vi "Version_4.9_8_on-chip_valves_for25ulSyringe_withModfied_Plunging.vi"() -> ()   [LabVIEW 2020] (continued)
                                n7542 = call "HardStopCurrentProcess (SubVI).vi"("VISA Refnum in"=w7985) -> ()  [unwired: 11 in]
                                }
                              }
                              n7543 = call "ProcessCompletionWaiter (SubVI).vi"("VISA Refnum in"=w7984) -> ()  [unwired: 11 in]
                            }
                            frame #4 {
                              # "Switch to Port-1"
                              # "Port-1 of the pump is conncted to Waste"
                              n7544 = local read "VISA Refnum in\nfor Pump"() -> (w7987:refnum<visa-resource-name>)
                              n7545 = call "PortChanger (SubVI).vi"("Port Number"="1", "VISA Refnum in"=w7987) -> ()  [unwired: 10 in]
                            }
                            frame #5 {
                              n7546 = local read "Stopper that ends \nthe main loops"() -> (w7988:bool)
                              n7547 = local read "VISA Refnum in\nfor Pump"() -> (w7989:refnum<visa-resource-name>)
                              n7548 = case shown="True" w7988 {
                                frame False {
                                }
                                frame True {
                                n7549 = local read "VISA Refnum in\nfor Pump"() -> (w7990:refnum<visa-resource-name>)
                                n7550 = call "HardStopCurrentProcess (SubVI).vi"("VISA Refnum in"=w7990) -> ()  [unwired: 11 in]
                                }
                              }
                              n7551 = call "ProcessCompletionWaiter (SubVI).vi"("VISA Refnum in"=w7989) -> ()  [unwired: 11 in]
                            }
                            frame #6 {
                              n7552 = local read "VISA Refnum in\nfor Pump"() -> (w7995:refnum<visa-resource-name>)
                              n7553 = local read "Volume of Syringe"() -> (w7994:dbl)
                              n7554 = call "GoToAbsolutePosition(SubVI).vi"("Absolute Volume Position in Syringe (in ul)"=0.0 ("Volume to be Dispensed"), "Volume of Syringe"=w7994, "Resolution of Pumping"=T2."Standard Pumping" ("Resolution for Dispensing"), "Flow Rate (ul/min)"=150.0 ("Dispense Flow Rate (ul/min)"), "VISA Refnum in"=w7995) -> ()  [unwired: 6 in, 1 out]
                            }
                            frame #7 {
                              n7555 = local read "Stopper that ends \nthe main loops"() -> (w7997:bool)
                              n7556 = case shown="True" w7997 {
                                frame False {
                                }
                                frame True {
                                n7557 = local read "VISA Refnum in\nfor Pump"() -> (w7998:refnum<visa-resource-name>)
                                n7558 = call "HardStopCurrentProcess (SubVI).vi"("VISA Refnum in"=w7998) -> ()  [unwired: 11 in]
                                }
                              }
                              n7559 = local read "VISA Refnum in\nfor Pump"() -> (w7996:refnum<visa-resource-name>)
                              n7560 = call "ProcessCompletionWaiter (SubVI).vi"("VISA Refnum in"=w7996) -> ()  [unwired: 11 in]
                            }
                          }
                        }
                      }
                      frame #1 {
                        n7561 = local read "No. of \ncleaning cycles"() -> (w7999:i32)
                        n7562 = for {
                          N: w7999 -> [_]
                          n7563 = stacked-sequence {
                            frame #0 {
                              # "Switch to Port-4"
                              # "Port-4 of pump is connected to Buffer-A"
                              n7564 = local read "VISA Refnum in\nfor Pump"() -> (w8002:refnum<visa-resource-name>)
                              n7565 = local write "Pause Data Collection"(TRUE ("Pause Data Collection")) -> ()
                              n7566 = call "PortChanger (SubVI).vi"("Port Number"="4", "VISA Refnum in"=w8002) -> ()  [unwired: 10 in]
                            }
                            frame #1 {
                              n7567 = local read "VISA Refnum in\nfor Pump"() -> (w8003:refnum<visa-resource-name>)
                              n7568 = call "ProcessCompletionWaiter (SubVI).vi"("VISA Refnum in"=w8003) -> ()  [unwired: 11 in]
                            }
                            frame #2 {
                              n7569 = local read "VISA Refnum in\nfor Pump"() -> (w8008:refnum<visa-resource-name>)
                              n7570 = local read "Apparent Volume\nof Syringe"() -> (w8004:dbl)
                              n7571 = local read "Volume of Syringe"() -> (w8007:dbl)
                              n7572 = call "RPickUp(SubVI).vi"("Volume to be picked up"=w8004, "Volume of Syringe"=w8007, "Resolution of PickUP"=T2."Standard Pumping", "PickUp Flow Rate (ul/min)"=150.0, "VISA Refnum in"=w8008) -> ()  [unwired: 6 in, 1 out]
                            }
                            frame #3 {
                              n7573 = local read "Stopper that ends \nthe main loops"() -> (w8009:bool)
                              n7574 = local read "VISA Refnum in\nfor Pump"() -> (w8010:refnum<visa-resource-name>)
                              n7575 = case shown="True" w8009 {
                                frame False {
                                }
                                frame True {
                                n7576 = local read "VISA Refnum in\nfor Pump"() -> (w8011:refnum<visa-resource-name>)
                                n7577 = call "HardStopCurrentProcess (SubVI).vi"("VISA Refnum in"=w8011) -> ()  [unwired: 11 in]
                                }
                              }
                              n7578 = call "ProcessCompletionWaiter (SubVI).vi"("VISA Refnum in"=w8010) -> ()  [unwired: 11 in]
                            }
                            frame #4 {
                              # "Switch to Port-1"
                              # "Port-1 of the pump is conncted to Waste"
                              n7579 = local read "VISA Refnum in\nfor Pump"() -> (w8013:refnum<visa-resource-name>)
                              n7580 = call "PortChanger (SubVI).vi"("Port Number"="1", "VISA Refnum in"=w8013) -> ()  [unwired: 10 in]
                            }
                            frame #5 {
                              n7581 = local read "Stopper that ends \nthe main loops"() -> (w8014:bool)
                              n7582 = local read "VISA Refnum in\nfor Pump"() -> (w8015:refnum<visa-resource-name>)
                              n7583 = case shown="True" w8014 {
                                frame False {
                                }
                                frame True {
                                n7584 = local read "VISA Refnum in\nfor Pump"() -> (w8016:refnum<visa-resource-name>)
                                n7585 = call "HardStopCurrentProcess (SubVI).vi"("VISA Refnum in"=w8016) -> ()  [unwired: 11 in]
                                }
                              }
                              n7586 = call "ProcessCompletionWaiter (SubVI).vi"("VISA Refnum in"=w8015) -> ()  [unwired: 11 in]
                            }
                            frame #6 {
                              n7587 = local read "VISA Refnum in\nfor Pump"() -> (w8021:refnum<visa-resource-name>)
                              n7588 = local read "Volume of Syringe"() -> (w8020:dbl)
                              n7589 = call "GoToAbsolutePosition(SubVI).vi"("Absolute Volume Position in Syringe (in ul)"=0.0 ("Volume to be Dispensed"), "Volume of Syringe"=w8020, "Resolution of Pumping"=T2."Standard Pumping" ("Resolution for Dispensing"), "Flow Rate (ul/min)"=150.0 ("Dispense Flow Rate (ul/min)"), "VISA Refnum in"=w8021) -> ()  [unwired: 6 in, 1 out]
                            }
                            frame #7 {
                              n7590 = local read "Stopper that ends \nthe main loops"() -> (w8023:bool)
                              n7591 = case shown="True" w8023 {
                                frame False {
                                }
                                frame True {
                                n7592 = local read "VISA Refnum in\nfor Pump"() -> (w8024:refnum<visa-resource-name>)
                                n7593 = call "HardStopCurrentProcess (SubVI).vi"("VISA Refnum in"=w8024) -> ()  [unwired: 11 in]
                                }
                              }
                              n7594 = local read "VISA Refnum in\nfor Pump"() -> (w8022:refnum<visa-resource-name>)
                              n7595 = call "ProcessCompletionWaiter (SubVI).vi"("VISA Refnum in"=w8022) -> ()  [unwired: 11 in]
                            }
                          }
                        }
                      }
                      frame #2 {
                        n7596 = local read "No. of \ncleaning cycles"() -> (w8025:i32)
                        n7597 = for {
                          N: w8025 -> [_]
                          n7598 = stacked-sequence {
                            frame #0 {
                              # "Switch to Port-4"
                              # "Port-4 of pump is connected to Buffer-A"
                              n7599 = local read "VISA Refnum in\nfor Pump"() -> (w8028:refnum<visa-resource-name>)
                              n7600 = local write "Pause Data Collection"(TRUE ("Pause Data Collection")) -> ()
                              n7601 = call "PortChanger (SubVI).vi"("Port Number"="5", "VISA Refnum in"=w8028) -> ()  [unwired: 10 in]
                            }
                            frame #1 {
                              n7602 = local read "VISA Refnum in\nfor Pump"() -> (w8029:refnum<visa-resource-name>)
                              n7603 = call "ProcessCompletionWaiter (SubVI).vi"("VISA Refnum in"=w8029) -> ()  [unwired: 11 in]
                            }
                            frame #2 {
                              n7604 = local read "VISA Refnum in\nfor Pump"() -> (w8034:refnum<visa-resource-name>)
                              n7605 = local read "Apparent Volume\nof Syringe"() -> (w8030:dbl)
                              n7606 = local read "Volume of Syringe"() -> (w8033:dbl)
                              n7607 = call "RPickUp(SubVI).vi"("Volume to be picked up"=w8030, "Volume of Syringe"=w8033, "Resolution of PickUP"=T2."Standard Pumping", "PickUp Flow Rate (ul/min)"=150.0, "VISA Refnum in"=w8034) -> ()  [unwired: 6 in, 1 out]
                            }
                            frame #3 {
                              n7608 = local read "Stopper that ends \nthe main loops"() -> (w8035:bool)
                              n7609 = local read "VISA Refnum in\nfor Pump"() -> (w8036:refnum<visa-resource-name>)
                              n7610 = case shown="True" w8035 {
                                frame False {
                                }
                                frame True {
                                n7611 = local read "VISA Refnum in\nfor Pump"() -> (w8037:refnum<visa-resource-name>)
                                n7612 = call "HardStopCurrentProcess (SubVI).vi"("VISA Refnum in"=w8037) -> ()  [unwired: 11 in]
                                }
                              }
                              n7613 = call "ProcessCompletionWaiter (SubVI).vi"("VISA Refnum in"=w8036) -> ()  [unwired: 11 in]
                            }
                            frame #4 {
                              # "Switch to Port-1"
                              # "Port-1 of the pump is conncted to Waste"
                              n7614 = local read "VISA Refnum in\nfor Pump"() -> (w8039:refnum<visa-resource-name>)
                              n7615 = call "PortChanger (SubVI).vi"("Port Number"="1", "VISA Refnum in"=w8039) -> ()  [unwired: 10 in]
                            }
                            frame #5 {
                              n7616 = local read "Stopper that ends \nthe main loops"() -> (w8040:bool)
                              n7617 = local read "VISA Refnum in\nfor Pump"() -> (w8041:refnum<visa-resource-name>)
                              n7618 = case shown="True" w8040 {
                                frame False {
                                }
                                frame True {
                                n7619 = local read "VISA Refnum in\nfor Pump"() -> (w8042:refnum<visa-resource-name>)
                                n7620 = call "HardStopCurrentProcess (SubVI).vi"("VISA Refnum in"=w8042) -> ()  [unwired: 11 in]
                                }
                              }
                              n7621 = call "ProcessCompletionWaiter (SubVI).vi"("VISA Refnum in"=w8041) -> ()  [unwired: 11 in]
                            }
                            frame #6 {
                              n7622 = local read "VISA Refnum in\nfor Pump"() -> (w8047:refnum<visa-resource-name>)
                              n7623 = local read "Volume of Syringe"() -> (w8046:dbl)
                              n7624 = call "GoToAbsolutePosition(SubVI).vi"("Absolute Volume Position in Syringe (in ul)"=0.0 ("Volume to be Dispensed"), "Volume of Syringe"=w8046, "Resolution of Pumping"=T2."Standard Pumping" ("Resolution for Dispensing"), "Flow Rate (ul/min)"=150.0 ("Dispense Flow Rate (ul/min)"), "VISA Refnum in"=w8047) -> ()  [unwired: 6 in, 1 out]
                            }
                            frame #7 {
                              n7625 = local read "Stopper that ends \nthe main loops"() -> (w8049:bool)
                              n7626 = case shown="True" w8049 {
                                frame False {
                                }
                                frame True {
                                n7627 = local read "VISA Refnum in\nfor Pump"() -> (w8050:refnum<visa-resource-name>)
                                n7628 = call "HardStopCurrentProcess (SubVI).vi"("VISA Refnum in"=w8050) -> ()  [unwired: 11 in]
                                }
                              }
                              n7629 = local read "VISA Refnum in\nfor Pump"() -> (w8048:refnum<visa-resource-name>)
                              n7630 = call "ProcessCompletionWaiter (SubVI).vi"("VISA Refnum in"=w8048) -> ()  [unwired: 11 in]
                            }
                          }
                        }
                      }
                      frame #3 {
                        n7631 = local read "No. of \ncleaning cycles"() -> (w8051:i32)
                        n7632 = for {
                          N: w8051 -> [_]
                          n7633 = stacked-sequence {
                            frame #0 {
                              # "Switch to Port-4"
                              # "Port-4 of pump is connected to Buffer-A"
                              n7634 = local read "VISA Refnum in\nfor Pump"() -> (w8054:refnum<visa-resource-name>)
                              n7635 = local write "Pause Data Collection"(TRUE ("Pause Data Collection")) -> ()
                              n7636 = call "PortChanger (SubVI).vi"("Port Number"="7", "VISA Refnum in"=w8054) -> ()  [unwired: 10 in]
                            }
                            frame #1 {
                              n7637 = local read "VISA Refnum in\nfor Pump"() -> (w8055:refnum<visa-resource-name>)
                              n7638 = call "ProcessCompletionWaiter (SubVI).vi"("VISA Refnum in"=w8055) -> ()  [unwired: 11 in]
                            }
                            frame #2 {
                              n7639 = local read "VISA Refnum in\nfor Pump"() -> (w8060:refnum<visa-resource-name>)
                              n7640 = local read "Apparent Volume\nof Syringe"() -> (w8056:dbl)
                              n7641 = local read "Volume of Syringe"() -> (w8059:dbl)
                              n7642 = call "RPickUp(SubVI).vi"("Volume to be picked up"=w8056, "Volume of Syringe"=w8059, "Resolution of PickUP"=T2."Standard Pumping", "PickUp Flow Rate (ul/min)"=150.0, "VISA Refnum in"=w8060) -> ()  [unwired: 6 in, 1 out]
                            }
                            frame #3 {
                              n7643 = local read "Stopper that ends \nthe main loops"() -> (w8061:bool)
                              n7644 = local read "VISA Refnum in\nfor Pump"() -> (w8062:refnum<visa-resource-name>)
                              n7645 = case shown="True" w8061 {
                                frame False {
                                }
                                frame True {
                                n7646 = local read "VISA Refnum in\nfor Pump"() -> (w8063:refnum<visa-resource-name>)
                                n7647 = call "HardStopCurrentProcess (SubVI).vi"("VISA Refnum in"=w8063) -> ()  [unwired: 11 in]
                                }
                              }
                              n7648 = call "ProcessCompletionWaiter (SubVI).vi"("VISA Refnum in"=w8062) -> ()  [unwired: 11 in]
                            }
                            frame #4 {
                              # "Switch to Port-1"
                              # "Port-1 of the pump is conncted to Waste"
                              n7649 = local read "VISA Refnum in\nfor Pump"() -> (w8065:refnum<visa-resource-name>)
                              n7650 = call "PortChanger (SubVI).vi"("Port Number"="1", "VISA Refnum in"=w8065) -> ()  [unwired: 10 in]
                            }
                            frame #5 {
                              n7651 = local read "Stopper that ends \nthe main loops"() -> (w8066:bool)
                              n7652 = local read "VISA Refnum in\nfor Pump"() -> (w8067:refnum<visa-resource-name>)
                              n7653 = case shown="True" w8066 {
                                frame False {
                                }
                                frame True {
                                n7654 = local read "VISA Refnum in\nfor Pump"() -> (w8068:refnum<visa-resource-name>)
                                n7655 = call "HardStopCurrentProcess (SubVI).vi"("VISA Refnum in"=w8068) -> ()  [unwired: 11 in]
                                }
                              }
                              n7656 = call "ProcessCompletionWaiter (SubVI).vi"("VISA Refnum in"=w8067) -> ()  [unwired: 11 in]
                            }
                            frame #6 {
                              n7657 = local read "VISA Refnum in\nfor Pump"() -> (w8073:refnum<visa-resource-name>)
                              n7658 = local read "Volume of Syringe"() -> (w8072:dbl)
                              n7659 = call "GoToAbsolutePosition(SubVI).vi"("Absolute Volume Position in Syringe (in ul)"=0.0 ("Volume to be Dispensed"), "Volume of Syringe"=w8072, "Resolution of Pumping"=T2."Standard Pumping" ("Resolution for Dispensing"), "Flow Rate (ul/min)"=150.0 ("Dispense Flow Rate (ul/min)"), "VISA Refnum in"=w8073) -> ()  [unwired: 6 in, 1 out]
                            }
                            frame #7 {
                              n7660 = local read "Stopper that ends \nthe main loops"() -> (w8075:bool)
                              n7661 = case shown="True" w8075 {
                                frame False {
                                }
                                frame True {
                                n7662 = local read "VISA Refnum in\nfor Pump"() -> (w8076:refnum<visa-resource-name>)
                                n7663 = call "HardStopCurrentProcess (SubVI).vi"("VISA Refnum in"=w8076) -> ()  [unwired: 11 in]
                                }
                              }
                              n7664 = local read "VISA Refnum in\nfor Pump"() -> (w8074:refnum<visa-resource-name>)
                              n7665 = call "ProcessCompletionWaiter (SubVI).vi"("VISA Refnum in"=w8074) -> ()  [unwired: 11 in]
                            }
                          }
                        }
                      }
                      frame #4 {
                        n7666 = local write "Start the Process"(FALSE ("Start the Process")) -> ()
                      }
                    }
                  }
                }
              }
              frame True {
                n7667 = local write "Pause Data Collection"(FALSE ("Pause Data Collection")) -> ()
              }
            }
          }
          frame "Check_Suction_Valve_functionality" {
            n7668 = local read "Start the Process"() -> (w8079:bool)
            n7669 = case shown="True" w8079 {
              frame False {
              }
              frame True {
                n7670 = while {
                  stop <- w8082 stop-if-true
                  n7671 = local read "Suction On/Off"() -> (w8080:bool)
                  n7672 = case shown="True" w8080 {
                    frame False {
                    }
                    frame True {
                      n7673 = stacked-sequence {
                        frame #0 {
                          n7674 = while {
                            stop <- w8083 stop-if-true
                            n7675 = local read "Stop for End of \nExperiment \nand Data Writing"() -> (w8085:bool)
                            n7676 = local read "Suction Pressure\nfor EM-grid \nDeposition (mbar)"() -> (w8088:sgl)
                            n7677 = local read "Suction On/Off"() -> (w8086:bool)
                            n7678 = call <vilib>:"fgt set pressure.vi"("pressure"=w8088, "pressureIndex"=u32 1) -> ()  [unwired: 9 in, 1 out]
                            n7679 = Not(x=w8086) -> (.not. x?=w8084:bool)
                            n7680 = Or(x=w8084, y=w8085) -> (x .or. y?=w8083:bool)
                            n7681 = Wait (ms)(milliseconds to wait=u32 100) -> ()  [unwired: 1 out]
                          }
                        }
                        frame #1 {
                          n7682 = for {
                            N: 2 -> [_]
                            n7683 = while {
                              stop <- w8093 stop-if-true
                              n7684 = local read "Stop for End of \nExperiment \nand Data Writing"() -> (w8095:bool)
                              n7685 = local read "Suction On/Off"() -> (w8096:bool)
                              n7686 = call <vilib>:"fgt set pressure.vi"("pressure"=sgl 0.0, "pressureIndex"=u32 1) -> ()  [unwired: 9 in, 1 out]
                              n7687 = Not(x=w8096) -> (.not. x?=w8094:bool)
                              n7688 = Or(x=w8094, y=w8095) -> (x .or. y?=w8093:bool)
                              n7689 = Wait (ms)(milliseconds to wait=u32 100) -> ()  [unwired: 1 out]
                            }
                            n7690 = Wait (ms)(milliseconds to wait=u32 400) -> ()  [unwired: 1 out]
                          }
                        }
                      }
                    }
                  }
                  n7691 = local read "Stop for End of \nExperiment \nand Data Writing"() -> (w8082:bool)
                  n7692 = Wait (ms)(milliseconds to wait=u32 100) -> ()  [unwired: 1 out]
                }
              }
            }
          }
          frame "Automated Plunging alone using purified protein from SEC column" {
            n7693 = local read "Stopper that ends \nthe main loops"() -> (w8099:bool)
            n7694 = case shown="False" w8099 {
              frame False {
                n7695 = local read "Start the Process"() -> (w8100:bool)
                n7696 = case shown="True" w8100 {
                  frame False {
                    n7697 = local read "Stopper that ends \nthe main loops"() -> (w8102:bool)
                    n7698 = local read "Start the Process"() -> (w8101:bool)
                    n7699 = Or(x=w8102, y=w8101) -> (x .or. y?=w8103:bool)
                    n7700 = case shown="False" w8103 {
                      frame False {
                        n7701 = while {
                          stop <- w8106 stop-if-true
                          n7702 = local read "Stop for End of \nExperiment \nand Data Writing"() -> (w8105:bool)
                          n7703 = local read "Stopper that ends \nthe main loops"() -> (w8108:bool)
                          n7704 = local read "Start the Process"() -> (w8107:bool)
                          n7705 = Wait (ms)(milliseconds to wait=u32 10) -> ()  [unwired: 1 out]
                          n7706 = Or(x=w8108, y=w8107) -> (x .or. y?=w8106:bool)
                          n7707 = local write "Stopper that ends \nthe main loops"(w8105) -> ()
                        }
                        n7708 = One Button Dialog(message="Please Select the Process and Press 'Start the Process' Button") -> ()  [unwired: 1 in, 1 out]
                      }
                      frame True {
                      }
                    }
                  }
                  frame True {
                    # "Elute Column-1, Divert Sample into Column-2, Elute column-2 and Divert the sample onto Grid"
                    n7709 = stacked-sequence {
                      frame #0 {
                        # "Sets suction pressure to zeros"
                        # "Switch to Port-5/8"
                        # "Port-5/8 of pump is connected to Buffer-C1/C2"
                        n7710 = local read "VISA Refnum in\nfor Pump"() -> (w8122:refnum<visa-resource-name>)
                        n7711 = Wait (ms)(milliseconds to wait=u32 500) -> ()  [unwired: 1 out]
                        n7712 = local write "Pause Data Collection"(TRUE ("Pause Data Collection")) -> ()
                        n7713 = local read "Port for \nC2-Elution"() -> (w8117:string)
                        n7714 = call "PortChanger (SubVI).vi"("Port Number"=w8117, "VISA Refnum in"=w8122) -> ()  [unwired: 10 in]
                        n7715 = local write "Valve V1 Open"(FALSE ("Valve V1 Open")) -> ()
                        n7716 = local write "Valve V2 Open"(FALSE ("Valve V2 Open")) -> ()
                        n7717 = local write "Valve V3 Open"(FALSE ("Valve V3 Open")) -> ()
                        n7718 = local write "Valve V4 Open"(FALSE ("Valve V4 Open")) -> ()
                        n7719 = local write "External Valve \nOpen"(FALSE ("External Valve \nOpen")) -> ()
                        n7720 = local write "Valve V8 Open"(FALSE ("Valve V8 Open")) -> ()
                        n7721 = local write "Valve V5 Open"(FALSE ("Valve V5 Open")) -> ()
                        n7722 = local write "Valve V6 Open"(FALSE ("Valve V6 Open")) -> ()
                        n7723 = local write "Valve V7 Open"(FALSE ("Valve V7 Open")) -> ()
                        n7724 = call <vilib>:"fgt set pressure.vi"("pressure"=sgl 0.0, "pressureIndex"=u32 1) -> ()  [unwired: 9 in, 1 out]
                      }
                      frame #1 {
                        n7725 = local read "VISA Refnum in\nfor Pump"() -> (w8126:refnum<visa-resource-name>)
                        n7726 = call "ProcessCompletionWaiter (SubVI).vi"("VISA Refnum in"=w8126) -> ()  [unwired: 11 in]
                        n7727 = local write "Start the Process"(FALSE ("Start the Process")) -> ()
                      }
                      frame #2 {
                        n7728 = local write "Elution of Column-1"(FALSE ("Elution of Column-1")) -> ()
                        n7729 = local write "Volume being Injected \nin this process"(0.0 ("Volume being Injected \nin this process")) -> ()
                        n7730 = local write "Elution of Column-2"(TRUE ("Elution of Column-2")) -> ()
                      }
                      frame #3 {
                        # "If Yes, it will clean the SEC buffer from port-8 tubing else it will clean the pump valve a bit"
                        n7731 = local read "Clean the \nBuffer-C2 tubing"() -> (w8130:bool)
                        n7732 = case shown="False" w8130 {
                          frame False {
                            n7733 = stacked-sequence {
                              frame #0 {
                                n7734 = local read "VISA Refnum in\nfor Pump"() -> (w8132:refnum<visa-resource-name>)
                                n7735 = local read "Port for \nC2-Elution"() -> (w8131:string)
                                n7736 = call "PortChanger (SubVI).vi"("Port Number"=w8131, "VISA Refnum in"=w8132) -> ()  [unwired: 10 in]
                              }
                              frame #1 {
                                n7737 = local read "VISA Refnum in\nfor Pump"() -> (w8133:refnum<visa-resource-name>)
                                n7738 = call "ProcessCompletionWaiter (SubVI).vi"("VISA Refnum in"=w8133) -> ()  [unwired: 11 in]
                              }
                              frame #2 {
                                n7739 = local read "Buffer-C2 Pumping\nResolution"() -> (w8136:T2)
                                n7740 = local read "VISA Refnum in\nfor Pump"() -> (w8138:refnum<visa-resource-name>)
                                n7741 = local read "V-S"() -> (w8134:dbl)
                                n7742 = local read "Volume of Syringe"() -> (w8137:dbl)
                                n7743 = call "RPickUp(SubVI).vi"("Volume to be picked up"=w8134, "Volume of Syringe"=w8137, "Resolution of PickUP"=w8136, "PickUp Flow Rate (ul/min)"=150.0, "VISA Refnum in"=w8138) -> ()  [unwired: 6 in, 1 out]
                              }
                              frame #3 {
                                n7744 = local read "Stopper that ends \nthe main loops"() -> (w8139:bool)
                                n7745 = local read "VISA Refnum in\nfor Pump"() -> (w8140:refnum<visa-resource-name>)
                                n7746 = case shown="True" w8139 {
                                frame False {
                                }
                                frame True {
                                n7747 = local read "VISA Refnum in\nfor Pump"() -> (w8141:refnum<visa-resource-name>)
                                n7748 = call "HardStopCurrentProcess (SubVI).vi"("VISA Refnum in"=w8141) -> ()  [unwired: 11 in]
                                }
                                }
                                n7749 = call "ProcessCompletionWaiter (SubVI).vi"("VISA Refnum in"=w8140) -> ()  [unwired: 11 in]
                              }
                              frame #4 {
                                n7750 = local read "VISA Refnum in\nfor Pump"() -> (w8143:refnum<visa-resource-name>)
                                n7751 = call "PortChanger (SubVI).vi"("Port Number"="1", "VISA Refnum in"=w8143) -> ()  [unwired: 10 in]
                              }
                              frame #5 {
                                n7752 = local read "Stopper that ends \nthe main loops"() -> (w8144:bool)
                                n7753 = local read "VISA Refnum in\nfor Pump"() -> (w8145:refnum<visa-resource-name>)
                                n7754 = case shown="True" w8144 {
                                frame False {
                                }
                                frame True {
                                n7755 = local read "VISA Refnum in\nfor Pump"() -> (w8146:refnum<visa-resource-name>)
                                n7756 = call "HardStopCurrentProcess (SubVI).vi"("VISA Refnum in"=w8146) -> ()  [unwired: 11 in]
                                }
                                }
                                n7757 = call "ProcessCompletionWaiter (SubVI).vi"("VISA Refnum in"=w8145) -> ()  [unwired: 11 in]
                              }
                              frame #6 {
                                n7758 = local read "VISA Refnum in\nfor Pump"() -> (w8151:refnum<visa-resource-name>)
                                n7759 = local read "Volume of Syringe"() -> (w8148:dbl)
                                n7760 = call "GoToAbsolutePosition(SubVI).vi"("Absolute Volume Position in Syringe (in ul)"=0.0, "Volume of Syringe"=w8148, "Resolution of Pumping"=T2."Standard Pumping", "Flow Rate (ul/min)"=150.0, "VISA Refnum in"=w8151) -> ()  [unwired: 6 in, 1 out]
                              }
                              frame #7 {
                                n7761 = local read "Stopper that ends \nthe main loops"() -> (w8152:bool)
                                n7762 = local read "VISA Refnum in\nfor Pump"() -> (w8153:refnum<visa-resource-name>)
                                n7763 = case shown="True" w8152 {
                                frame False {
                                }
                                frame True {
                                n7764 = local read "VISA Refnum in\nfor Pump"() -> (w8154:refnum<visa-resource-name>)
                                n7765 = call "HardStopCurrentProcess (SubVI).vi"("VISA Refnum in"=w8154) -> ()  [unwired: 11 in]
                                }
                                }
                                n7766 = call "ProcessCompletionWaiter (SubVI).vi"("VISA Refnum in"=w8153) -> ()  [unwired: 11 in]
                              }
                            }
                          }
                          frame True {
                            n7767 = for {
                              N: 2 -> [_]
                              n7768 = stacked-sequence {
                                frame #0 {
                                n7769 = local read "VISA Refnum in\nfor Pump"() -> (w8157:refnum<visa-resource-name>)
                                n7770 = local read "Port for \nC2-Elution"() -> (w8156:string)
                                n7771 = call "PortChanger (SubVI).vi"("Port Number"=w8156, "VISA Refnum in"=w8157) -> ()  [unwired: 10 in]
                                }
                                frame #1 {
                                n7772 = local read "VISA Refnum in\nfor Pump"() -> (w8158:refnum<visa-resource-name>)
                                n7773 = call "ProcessCompletionWaiter (SubVI).vi"("VISA Refnum in"=w8158) -> ()  [unwired: 11 in]
                                }
                                frame #2 {
                                n7774 = local read "Buffer-C2 Pumping\nResolution"() -> (w8161:T2)
                                n7775 = local read "VISA Refnum in\nfor Pump"() -> (w8163:refnum<visa-resource-name>)
                                n7776 = local read "Apparent Volume\nof Syringe"() -> (w8159:dbl)
                                n7777 = local read "Volume of Syringe"() -> (w8162:dbl)
                                n7778 = call "RPickUp(SubVI).vi"("Volume to be picked up"=w8159, "Volume of Syringe"=w8162, "Resolution of PickUP"=w8161, "PickUp Flow Rate (ul/min)"=150.0, "VISA Refnum in"=w8163) -> ()  [unwired: 6 in, 1 out]
                                }
                                frame #3 {
                                n7779 = local read "Stopper that ends \nthe main loops"() -> (w8164:bool)
                                n7780 = local read "VISA Refnum in\nfor Pump"() -> (w8165:refnum<visa-resource-name>)
                                n7781 = case shown="True" w8164 {
                                frame False {
                                }
                                frame True {
                                n7782 = local read "VISA Refnum in\nfor Pump"() -> (w8166:refnum<visa-resource-name>)
                                n7783 = call "HardStopCurrentProcess (SubVI).vi"("VISA Refnum in"=w8166) -> ()  [unwired: 11 in]
                                }
                                }
                                n7784 = call "ProcessCompletionWaiter (SubVI).vi"("VISA Refnum in"=w8165) -> ()  [unwired: 11 in]
                                }
                                frame #4 {
                                n7785 = local read "VISA Refnum in\nfor Pump"() -> (w8168:refnum<visa-resource-name>)
                                n7786 = call "PortChanger (SubVI).vi"("Port Number"="1", "VISA Refnum in"=w8168) -> ()  [unwired: 10 in]
                                }
                                frame #5 {
                                n7787 = local read "Stopper that ends \nthe main loops"() -> (w8169:bool)
                                n7788 = local read "VISA Refnum in\nfor Pump"() -> (w8170:refnum<visa-resource-name>)
                                n7789 = case shown="True" w8169 {
                                frame False {
                                }
                                frame True {
                                n7790 = local read "VISA Refnum in\nfor Pump"() -> (w8171:refnum<visa-resource-name>)
                                n7791 = call "HardStopCurrentProcess (SubVI).vi"("VISA Refnum in"=w8171) -> ()  [unwired: 11 in]
                                }
                                }
                                n7792 = call "ProcessCompletionWaiter (SubVI).vi"("VISA Refnum in"=w8170) -> ()  [unwired: 11 in]
                                }
                                frame #6 {
                                n7793 = local read "VISA Refnum in\nfor Pump"() -> (w8176:refnum<visa-resource-name>)
                                n7794 = local read "Volume of Syringe"() -> (w8173:dbl)
                                n7795 = call "GoToAbsolutePosition(SubVI).vi"("Absolute Volume Position in Syringe (in ul)"=0.0, "Volume of Syringe"=w8173, "Resolution of Pumping"=T2."Standard Pumping", "Flow Rate (ul/min)"=150.0, "VISA Refnum in"=w8176) -> ()  [unwired: 6 in, 1 out]
                                }
                                frame #7 {
                                n7796 = local read "Stopper that ends \nthe main loops"() -> (w8177:bool)
                                n7797 = local read "VISA Refnum in\nfor Pump"() -> (w8178:refnum<visa-resource-name>)
                                n7798 = case shown="True" w8177 {
                                frame False {
                                }
                                frame True {
                                n7799 = local read "VISA Refnum in\nfor Pump"() -> (w8179:refnum<visa-resource-name>)
                                n7800 = call "HardStopCurrentProcess (SubVI).vi"("VISA Refnum in"=w8179) -> ()  [unwired: 11 in]
                                }
                                }
                                n7801 = call "ProcessCompletionWaiter (SubVI).vi"("VISA Refnum in"=w8178) -> ()  [unwired: 11 in]
                                }
                              }
                            }
                          }
                        }
                      }
                      frame #4 {
                        n7802 = local read "VISA Refnum in\nfor Pump"() -> (w8181:refnum<visa-resource-name>)
                        n7803 = local read "Port for \nC2-Elution"() -> (w8180:string)
                        n7804 = call "PortChanger (SubVI).vi"("Port Number"=w8180, "VISA Refnum in"=w8181) -> ()  [unwired: 10 in]
                      }
                      frame #5 {
                        n7805 = local read "VISA Refnum in\nfor Pump"() -> (w8182:refnum<visa-resource-name>)
                        n7806 = call "ProcessCompletionWaiter (SubVI).vi"("VISA Refnum in"=w8182) -> ()  [unwired: 11 in]
                      }
                      frame #6 {
                        n7807 = local read "Buffer-C2 PickUp \nFlow Rate (ul/min)"() -> (w8186:dbl)
                        n7808 = local read "Buffer-C2 Pumping\nResolution"() -> (w8185:T2)
                        n7809 = local read "VISA Refnum in\nfor Pump"() -> (w8188:refnum<visa-resource-name>)
                        n7810 = local read "Buffer-C2 Volume \nto be Pumped"() -> (w8184:dbl)
                        n7811 = local read "Volume of Syringe"() -> (w8187:dbl)
                        n7812 = call "RPickUp(SubVI).vi"("Volume to be picked up"=w8184, "Volume of Syringe"=w8187, "Resolution of PickUP"=w8185, "PickUp Flow Rate (ul/min)"=w8186, "VISA Refnum in"=w8188) -> ()  [unwired: 6 in, 1 out]
                        n7813 = local write "SEC On"(TRUE ("SEC On")) -> ()
                      }
                      frame #7 {
                        n7814 = local read "Stopper that ends \nthe main loops"() -> (w8189:bool)
                        n7815 = local read "VISA Refnum in\nfor Pump"() -> (w8190:refnum<visa-resource-name>)
                        n7816 = case shown="True" w8189 {
                          frame False {
                          }
                          frame True {
                            n7817 = local read "VISA Refnum in\nfor Pump"() -> (w8191:refnum<visa-resource-name>)
                            n7818 = call "HardStopCurrentProcess (SubVI).vi"("VISA Refnum in"=w8191) -> ()  [unwired: 11 in]
                          }
                        }
                        n7819 = call "ProcessCompletionWaiter (SubVI).vi"("VISA Refnum in"=w8190) -> ()  [unwired: 11 in]
                      }
                      frame #8 {
                        # "Reads the initial Plunger Position for computing the volume dispensed"
                        n7820 = local read "VISA Refnum in\nfor Pump"() -> (w8193:refnum<visa-resource-name>)
                        n7821 = call "AbsolutePlungerPosition (SubVI).vi"("VISA Refnum in"=w8193) -> ("Plunger Position"=w8192:i32)  [unwired: 10 in]
                        n7822 = local write "Initial Plunger Position"(w8192) -> ()
                      }
                      frame #9 {
                        # "Switch to Port-10"
                        # "Port-10 of the pump is conncted to column-2 of chip"
                        n7823 = local read "VISA Refnum in\nfor Pump"() -> (w8195:refnum<visa-resource-name>)
                        n7824 = call "PortChanger (SubVI).vi"("Port Number"="10", "VISA Refnum in"=w8195) -> ()  [unwired: 10 in]
                      }
                      frame #10 {
                        n7825 = local read "Stopper that ends \nthe main loops"() -> (w8196:bool)
                        n7826 = local read "VISA Refnum in\nfor Pump"() -> (w8197:refnum<visa-resource-name>)
                        n7827 = call "ProcessCompletionWaiter (SubVI).vi"("VISA Refnum in"=w8197) -> ()  [unwired: 11 in]
                        n7828 = case shown="True" w8196 {
                          frame False {
                          }
                          frame True {
                            n7829 = local read "VISA Refnum in\nfor Pump"() -> (w8198:refnum<visa-resource-name>)
                            n7830 = call "HardStopCurrentProcess (SubVI).vi"("VISA Refnum in"=w8198) -> ()  [unwired: 11 in]
                          }
                        }
                      }
                      frame #11 {
                        # "Keeps the AMF valve after column-1 open and valve after column-2 closed"
                        n7831 = local read "Buffer-C2 Dispense\nFlow Rate (ul/min)"() -> (w8211:dbl)
                        n7832 = local read "Buffer-C2 Pumping\nResolution"() -> (w8210:T2)
                        n7833 = local read "VISA Refnum in\nfor Pump"() -> (w8213:refnum<visa-resource-name>)
                        n7834 = local write "Pause Data Collection"(FALSE ("Pause Data Collection")) -> ()
                        n7835 = local read "Volume of Syringe"() -> (w8212:dbl)
                        n7836 = call "GoToAbsolutePosition(SubVI).vi"("Absolute Volume Position in Syringe (in ul)"=0.0 ("Volume to be Dispensed"), "Volume of Syringe"=w8212, "Resolution of Pumping"=w8210, "Flow Rate (ul/min)"=w8211, "VISA Refnum in"=w8213) -> ()  [unwired: 6 in, 1 out]
                        n7837 = local write "Valve V1 Open"(FALSE ("Valve V1 Open")) -> ()
                        n7838 = local write "Valve V2 Open"(TRUE ("Valve V2 Open")) -> ()
                        n7839 = local write "Valve V3 Open"(TRUE ("Valve V3 Open")) -> ()
                        n7840 = local write "Valve V4 Open"(FALSE ("Valve V4 Open")) -> ()
                        n7841 = local write "External Valve \nOpen"(TRUE ("External Valve \nOpen")) -> ()
                        n7842 = local write "Valve V8 Open"(FALSE ("Valve V8 Open")) -> ()
                        n7843 = local write "Valve V5 Open"(FALSE ("Valve V5 Open")) -> ()
                        n7844 = local write "Valve V6 Open"(FALSE ("Valve V6 Open")) -> ()
                        n7845 = local write "Valve V7 Open"(FALSE ("Valve V7 Open")) -> ()
                      }
                      frame #12 {
                        n7846 = local read "Initial Plunger Position"() -> (w8217:dbl)
                        n7847 = local read "Buffer-C2 Pumping\nResolution"() -> (w8216:T2)
                        n7848 = local read "VISA Refnum in\nfor Pump"() -> (w8218:refnum<visa-resource-name>)
                        n7849 = local read "Volume of Syringe"() -> (w8215:dbl)
                        n7850 = while {
                          tunnel: w8217 -> [w8224]
                          tunnel: w8218 -> [w8223]
                          tunnel: w8216 -> [w8222]
                          tunnel: w8215 -> [w8221]
                          stop <- w8219 stop-if-true
                          n7851 = Wait (ms)(milliseconds to wait=u32 100) -> ()  [unwired: 1 out]
                          n7852 = stacked-sequence {
                            tunnel: w8224 -> [w8230 _]
                            tunnel: w8223 -> [w8229 w8256]
                            tunnel: w8222 -> [w8228 _]
                            tunnel: w8221 -> [w8227 _]
                            tunnel: [_ w8252] -> w8219
                            frame #0 {
                              n7853 = call "AbsolutePlungerPosition (SubVI).vi"("VISA Refnum in"=w8229) -> ("Plunger Position"=w8226:i32)  [unwired: 10 in]
                              n7854 = case shown="\"Standard Pumping\", Default" w8228 {
                                tunnel: w8230 -> [w8235 w8244]
                                tunnel: w8226 -> [w8236 w8243]
                                tunnel: [w8234 w8241] -> w8225
                                tunnel: w8227 -> [w8233 w8242]
                                frame "Standard Pumping", Default {
                                n7855 = Subtract(x=w8235, y=w8236) -> (x-y=w8232:dbl)
                                n7856 = Absolute Value(x=w8232) -> (abs(x)=w8231:dbl)
                                n7857 = Multiply(x=w8231, y=w8233) -> (x*y=w8238:dbl)
                                n7858 = Divide(x=w8238, y=3000.0) -> (x/y=w8234:dbl)
                                }
                                frame "High Resolution Pumping" {
                                n7859 = Subtract(x=w8244, y=w8243) -> (x-y=w8240:dbl)
                                n7860 = Absolute Value(x=w8240) -> (abs(x)=w8239:dbl)
                                n7861 = Multiply(x=w8239, y=w8242) -> (x*y=w8246:dbl)
                                n7862 = Divide(x=w8246, y=24000.0) -> (x/y=w8241:dbl)
                                }
                              }
                              n7863 = local write "Volume being Injected \nin this process"(w8225) -> ()
                            }
                            frame #1 {
                              n7864 = local read "Stopper that ends \nthe main loops"() -> (w8253:bool)
                              n7865 = local read "Divert Buffer-C \ninto Column-2"() -> (w8254:bool)
                              n7866 = local read "Volume being Injected \nin this process"() -> (w8251:dbl)
                              n7867 = call "LSPOneStatus (SubVI).vi"("VISA Refnum in"=w8256) -> ("read buffer"=w8258:string)  [unwired: 10 in]
                              n7868 = call <vilib>:"Trim Whitespace.vi"("string"=w8258) -> ("trimmed string"=w8257:string)  [unwired: 1 in]
                              n7869 = Equal?(x=w8257, y="/0`\u0003") -> (x = y?=w8255:bool)
                              n7870 = Or(x=w8254, y=w8253) -> (x .or. y?=w8249:bool)
                              n7871 = Greater Or Equal?(x=w8251, y=2.0) -> (x >= y?=w8248:bool)
                              n7872 = Or(x=w8249, y=w8248) -> (x .or. y?=w8247:bool)
                              n7873 = Or(x=w8255, y=w8247) -> (x .or. y?=w8252:bool)
                            }
                          }
                        }
                        n7874 = local read "Stopper that ends \nthe main loops"() -> (w8214:bool)
                        n7875 = case shown="True" w8214 {
                          frame False {
                          }
                          frame True {
                            n7876 = local read "VISA Refnum in\nfor Pump"() -> (w8260:refnum<visa-resource-name>)
                            n7877 = call "HardStopCurrentProcess (SubVI).vi"("VISA Refnum in"=w8260) -> ()  [unwired: 11 in]
                          }
                        }
                      }
                      frame #13 {
                        # "Keeps the on-chip valves V4, V5 and V7 open"
                        # "Keeps the AMF valve after column-1 closed and valve after column-2 open"
                        n7878 = local write "Divert Buffer-C \ninto Column-2"(FALSE ("Divert Buffer-C \ninto Column-2")) -> ()
                        n7879 = local write "Valve V3 Open"(TRUE ("Valve V3 Open")) -> ()
                        n7880 = local write "Valve V2 Open"(FALSE ("Valve V2 Open")) -> ()
                        n7881 = local write "Valve V1 Open"(FALSE ("Valve V1 Open")) -> ()
                        n7882 = local write "Valve V4 Open"(TRUE ("Valve V4 Open")) -> ()
                        n7883 = local write "External Valve \nOpen"(FALSE ("External Valve \nOpen")) -> ()
                        n7884 = local write "Valve V5 Open"(TRUE ("Valve V5 Open")) -> ()
                        n7885 = local write "Valve V6 Open"(FALSE ("Valve V6 Open")) -> ()
                        n7886 = local write "Valve V8 Open"(FALSE ("Valve V8 Open")) -> ()
                        n7887 = local write "Valve V7 Open"(TRUE ("Valve V7 Open")) -> ()
                      }
                      frame #14 {
                        n7888 = local read "Initial Plunger Position"() -> (w8274:dbl)
                        n7889 = local read "Buffer-C2 Pumping\nResolution"() -> (w8273:T2)
                        n7890 = local read "VISA Refnum in\nfor Pump"() -> (w8275:refnum<visa-resource-name>)
                        n7891 = local read "Volume of Syringe"() -> (w8272:dbl)
                        n7892 = while {
                          tunnel: w8274 -> [w8281]
                          tunnel: w8275 -> [w8280]
                          tunnel: w8273 -> [w8279]
                          tunnel: w8272 -> [w8278]
                          stop <- w8276 stop-if-true
                          n7893 = Wait (ms)(milliseconds to wait=u32 100) -> ()  [unwired: 1 out]
                          n7894 = stacked-sequence {
                            tunnel: w8281 -> [w8287 _]
                            tunnel: w8280 -> [w8286 w8309]
                            tunnel: w8279 -> [w8285 _]
                            tunnel: w8278 -> [w8284 _]
                            tunnel: [_ w8307] -> w8276
                            frame #0 {
                              n7895 = call "AbsolutePlungerPosition (SubVI).vi"("VISA Refnum in"=w8286) -> ("Plunger Position"=w8283:i32)  [unwired: 10 in]
                              n7896 = case shown="\"Standard Pumping\", Default" w8285 {
                                tunnel: w8287 -> [w8292 w8301]
                                tunnel: w8283 -> [w8293 w8300]
                                tunnel: [w8291 w8298] -> w8282
                                tunnel: w8284 -> [w8290 w8299]
                                frame "Standard Pumping", Default {
                                n7897 = Subtract(x=w8292, y=w8293) -> (x-y=w8289:dbl)
                                n7898 = Absolute Value(x=w8289) -> (abs(x)=w8288:dbl)
                                n7899 = Multiply(x=w8288, y=w8290) -> (x*y=w8295:dbl)
                                n7900 = Divide(x=w8295, y=3000.0) -> (x/y=w8291:dbl)
                                }
                                frame "High Resolution Pumping" {
                                n7901 = Subtract(x=w8301, y=w8300) -> (x-y=w8297:dbl)
                                n7902 = Absolute Value(x=w8297) -> (abs(x)=w8296:dbl)
                                n7903 = Multiply(x=w8296, y=w8299) -> (x*y=w8303:dbl)
                                n7904 = Divide(x=w8303, y=24000.0) -> (x/y=w8298:dbl)
                                }
                              }
                              n7905 = local write "Volume being Injected \nin this process"(w8282) -> ()
                            }
                            frame #1 {
                              n7906 = call "LSPOneStatus (SubVI).vi"("VISA Refnum in"=w8309) -> ("read buffer"=w8311:string)  [unwired: 10 in]
                              n7907 = call <vilib>:"Trim Whitespace.vi"("string"=w8311) -> ("trimmed string"=w8310:string)  [unwired: 1 in]
                              n7908 = Equal?(x=w8310, y="/0`\u0003") -> (x = y?=w8308:bool)
                              n7909 = local read "Stopper that ends \nthe main loops"() -> (w8305:bool)
                              n7910 = local read "Divert Sample \nonto Grid"() -> (w8306:bool)
                              n7911 = Or(x=w8306, y=w8305) -> (x .or. y?=w8304:bool)
                              n7912 = Or(x=w8308, y=w8304) -> (x .or. y?=w8307:bool)
                            }
                          }
                        }
                        n7913 = local read "Stopper that ends \nthe main loops"() -> (w8271:bool)
                        n7914 = case shown="True" w8271 {
                          frame False {
                          }
                          frame True {
                            n7915 = local read "VISA Refnum in\nfor Pump"() -> (w8313:refnum<visa-resource-name>)
                            n7916 = call "HardStopCurrentProcess (SubVI).vi"("VISA Refnum in"=w8313) -> ()  [unwired: 11 in]
                          }
                        }
                      }
                      frame #15 {
                        n7917 = local read "Volume being Injected \nin this process"() -> (w8316:dbl)
                        n7918 = local read "VISA Refnum in\nfor Pump"() -> (w8318:refnum<visa-resource-name>)
                        n7919 = call "AbsolutePlungerPosition (SubVI).vi"("VISA Refnum in"=w8318) -> ("Plunger Position"=w8317:i32)  [unwired: 10 in]
                        n7920 = local write "Pause Data Collection"(TRUE) -> ()
                        n7921 = local write "True Volume being \ninjected in this\nprocess"(w8316) -> ()
                        n7922 = local write "Position\nNow"(w8317) -> ()
                        n7923 = Wait (ms)(milliseconds to wait=u32 500) -> ()  [unwired: 1 out]
                      }
                      frame #16 {
                        # "Sample Deposition onto EM-Grid"
                        n7924 = local read "Divert Sample \nonto Grid"() -> (w8319:bool)
                        n7925 = case shown="True" w8319 {
                          frame False {
                          }
                          frame True {
                            n7926 = stacked-sequence {
                              frame #0 {
                                # "Discard the initial volume of fluid that is present in the channel prior to detection"
                                n7927 = local read "Buffer-C2 Pumping\nResolution"() -> (w8332:T2)
                                n7928 = local read "Initial Plunger Position"() -> (w8331:dbl)
                                n7929 = local read "VISA Refnum in\nfor Pump"() -> (w8333:refnum<visa-resource-name>)
                                n7930 = local read "Position\nNow"() -> (w8329:dbl)
                                n7931 = local read "Volume of Syringe"() -> (w8330:dbl)
                                n7932 = local write "Pause Data Collection"(FALSE) -> ()
                                n7933 = while {
                                tunnel: w8333 -> [w8343]
                                tunnel: w8332 -> [w8342]
                                tunnel: w8331 -> [w8338]
                                tunnel: w8330 -> [w8341]
                                tunnel: w8329 -> [w8337]
                                stop <- w8339 stop-if-true
                                n7934 = stacked-sequence {
                                tunnel: w8343 -> [w8349 w8371 w8403]
                                tunnel: w8342 -> [w8348 w8370 _]
                                tunnel: w8338 -> [w8346 _ _]
                                tunnel: w8341 -> [w8345 w8368 _]
                                tunnel: [_ _ w8397] -> w8339
                                tunnel: w8337 -> [_ w8366 _]
                                frame #0 {
                                # "From here on 'True Volume being injected \nin this process' represents the true total \nvolume in this process"
                                n7935 = call "AbsolutePlungerPosition (SubVI).vi"("VISA Refnum in"=w8349) -> ("Plunger Position"=w8347:i32)  [unwired: 10 in]
                                n7936 = case shown="..\"Standard Pumping\"" w8348 {
                                tunnel: w8347 -> [w8357 w8365]
                                tunnel: w8346 -> [w8356 w8364]
                                tunnel: w8345 -> [w8353 w8361]
                                tunnel: [w8350 w8358] -> w8344
                                frame .."Standard Pumping" {
                                n7937 = Subtract(x=w8357, y=w8356) -> (x-y=w8355:dbl)
                                n7938 = Absolute Value(x=w8355) -> (abs(x)=w8354:dbl)
                                n7939 = Multiply(x=w8354, y=w8353) -> (x*y=w8352:dbl)
                                n7940 = Divide(x=w8352, y=3000.0) -> (x/y=w8350:dbl)
                                }
                                frame "High Resolution Pumping".. {
                                n7941 = Subtract(x=w8365, y=w8364) -> (x-y=w8363:dbl)
                                n7942 = Absolute Value(x=w8363) -> (abs(x)=w8362:dbl)
                                n7943 = Multiply(x=w8362, y=w8361) -> (x*y=w8360:dbl)
                                n7944 = Divide(x=w8360, y=24000.0) -> (x/y=w8358:dbl)
                                }
                                }
                                n7945 = local write "True Volume being \ninjected in this\nprocess"(w8344) -> ()
                                }
                                frame #1 {
                                # "From here on 'Volume being injected \nin this process' represents the volume \nin this sub process"
                                n7946 = call "AbsolutePlungerPosition (SubVI).vi"("VISA Refnum in"=w8371) -> ("Plunger Position"=w8369:i32)  [unwired: 10 in]
                                n7947 = case shown="..\"Standard Pumping\"" w8370 {
                                tunnel: w8369 -> [w8379 w8387]
                                tunnel: w8366 -> [w8378 w8386]
                                tunnel: w8368 -> [w8375 w8383]
                                tunnel: [w8372 w8380] -> w8367
                                frame .."Standard Pumping" {
                                n7948 = Subtract(x=w8379, y=w8378) -> (x-y=w8377:dbl)
                                n7949 = Absolute Value(x=w8377) -> (abs(x)=w8376:dbl)
                                n7950 = Multiply(x=w8376, y=w8375) -> (x*y=w8374:dbl)
                                n7951 = Divide(x=w8374, y=3000.0) -> (x/y=w8372:dbl)
                                }
                                frame "High Resolution Pumping".. {
                                n7952 = Subtract(x=w8387, y=w8386) -> (x-y=w8385:dbl)
                                n7953 = Absolute Value(x=w8385) -> (abs(x)=w8384:dbl)
                                n7954 = Multiply(x=w8384, y=w8383) -> (x*y=w8382:dbl)
                                n7955 = Divide(x=w8382, y=24000.0) -> (x/y=w8380:dbl)
                                }
                                }
                                n7956 = local write "Volume being Injected \nin this process"(w8367) -> ()
                                }
                                frame #2 {
                                n7957 = local read "Discard Volume"() -> (w8391:dbl)
                                n7958 = local read "Discard fluid \nprior to 1st \ndeposition"() -> (w8396:bool)
                                n7959 = local read "Volume being Injected \nin this process"() -> (w8395:dbl)
                                n7960 = Greater Or Equal?(x=w8395, y=w8391) -> (x >= y?=w8393:bool)
                                n7961 = call "AbsolutePlungerPositionStatus (SubVI).vi"("VISA Refnum in"=w8403) -> ("read buffer"=w8402:string)  [unwired: 10 in]
                                n7962 = local read "Stop for End of \nExperiment \nand Data Writing"() -> (w8390:bool)
                                n7963 = call <vilib>:"Trim Whitespace.vi"("string"=w8402) -> ("trimmed string"=w8401:string)  [unwired: 1 in]
                                n7964 = Not(x=w8396) -> (.not. x?=w8394:bool)
                                n7965 = Equal?(x=w8401, y="/0`\u0003") -> (x = y?=w8399:bool)
                                n7966 = Or(x=w8394, y=w8393) -> (x .or. y?=w8392:bool)
                                n7967 = local read "Re-SEC"() -> (w8389:bool)
                                n7968 = Or(x=w8390, y=w8389) -> (x .or. y?=w8388:bool)
                                n7969 = Or(x=w8392, y=w8388) -> (x .or. y?=w8398:bool)
                                n7970 = Or(x=w8399, y=w8398) -> (x .or. y?=w8397:bool)
                                }
                                }
                                n7971 = Wait (ms)(milliseconds to wait=u32 100) -> ()  [unwired: 1 out]
                                }
                                n7972 = local write "Valve V4 Open"(TRUE ("Valve V4 Open")) -> ()
                                n7973 = local write "Valve V3 Open"(TRUE ("Valve V3 Open")) -> ()
                                n7974 = local write "Valve V2 Open"(FALSE ("Valve V2 Open")) -> ()
                                n7975 = local write "Valve V1 Open"(FALSE ("Valve V1 Open")) -> ()
                                n7976 = local write "External Valve \nOpen"(FALSE ("External Valve \nOpen")) -> ()
                                n7977 = local write "Valve V5 Open"(TRUE ("Valve V5 Open")) -> ()
                                n7978 = local write "Valve V6 Open"(TRUE ("Valve V6 Open")) -> ()
                                n7979 = local write "Valve V8 Open"(FALSE ("Valve V8 Open")) -> ()
                                n7980 = local write "Valve V7 Open"(FALSE ("Valve V7 Open")) -> ()
                                n7981 = local write "Volume being Injected \nin this process"(0.0) -> ()
                              }
                              frame #1 {
                                # "Keeps the on-chip valve V1, V2 and V3 closed,\nHalts also deposition onto the grid\nand waits for the 1st redeposit command. Once the command is issued\nit starts pumpoing and moves onto the next frame"
                                n7982 = stacked-sequence {
                                frame #0 {
                                n7983 = local write "Valve V5 Open"(FALSE ("Valve V5 Open")) -> ()
                                n7984 = local write "Valve V1 Open"(FALSE ("Valve V1 Open")) -> ()
                                n7985 = local read "VISA Refnum in\nfor Pump"() -> (w8415:refnum<visa-resource-name>)
                                n7986 = local write "Valve V2 Open"(FALSE ("Valve V2 Open")) -> ()
                                n7987 = local write "Valve V6 Open"(FALSE ("Valve V6 Open")) -> ()
                                n7988 = local write "Re-deposit Sample\nonto Grid"(FALSE ("Redeposit Sample\nonto Grid")) -> ()
                                n7989 = local write "Pause Data Collection"(TRUE ("Pause Data Collection")) -> ()
                                n7990 = call "HardStopCurrentProcess (SubVI).vi"("VISA Refnum in"=w8415) -> ()  [unwired: 11 in]
                                n7991 = local write "Valve V7 Open"(FALSE ("Valve V7 Open")) -> ()
                                n7992 = local write "Valve V3 Open"(FALSE ("Valve V3 Open")) -> ()
                                n7993 = local write "External Valve \nOpen"(FALSE ("External Valve \nOpen")) -> ()
                                n7994 = local write "Valve V4 Open"(FALSE ("Valve V4 Open")) -> ()
                                n7995 = local write "Valve V8 Open"(FALSE ("Valve V8 Open")) -> ()
                                }
                                frame #1 {
                                n7996 = while {
                                stop <- w8421 stop-if-true
                                n7997 = local read "Stop for End of \nExperiment \nand Data Writing"() -> (w8419:bool)
                                n7998 = local read "Re-SEC"() -> (w8420:bool)
                                n7999 = local read "Re-deposit Sample\nonto Grid"() -> (w8422:bool)
                                n8000 = Or(x=w8419, y=w8420) -> (x .or. y?=w8418:bool)
                                n8001 = Or(x=w8422, y=w8418) -> (x .or. y?=w8421:bool)
                                }
                                n8002 = local write "Discard fluid \nprior to 1st \ndeposition"(FALSE ("Discard fluid \nprior to 1st \ndeposition")) -> ()
                                n8003 = One Button Dialog(message="Do you want to deposit sample on another grid? If yes, turn on 'Re-deposit Sample onto Grid'. Else turn on Re-SEC to do SEC again or STOP to end the experiment") -> ()  [unwired: 1 in, 1 out]
                                }
                                frame #2 {
                                n8004 = local write "Valve V6 Open"(TRUE ("Valve V3 Open")) -> ()
                                n8005 = local write "Valve V4 Open"(TRUE ("Valve V1 Open")) -> ()
                                n8006 = local write "Valve V5 Open"(TRUE ("Valve V2 Open")) -> ()
                                n8007 = local write "Valve V3 Open"(TRUE ("Valve V3 Open")) -> ()
                                n8008 = local write "Valve V7 Open"(FALSE ("Valve V7 Open")) -> ()
                                }
                                frame #3 {
                                n8009 = local read "Re-deposit Sample\nonto Grid"() -> (w8428:bool)
                                n8010 = case shown="True" w8428 {
                                frame False {
                                n8011 = local write "Suction On/Off"(FALSE ("Suction On/Off")) -> ()
                                }
                                frame True {
                                n8012 = stacked-sequence {
                                frame #0 {
                                n8013 = local read "VISA Refnum in\nfor Pump"() -> (w8431:refnum<visa-resource-name>)
                                n8014 = call "AbsolutePlungerPosition (SubVI).vi"("VISA Refnum in"=w8431) -> ("Plunger Position"=w8430:i32)  [unwired: 10 in]
                                n8015 = local write "Position\nNow"(w8430) -> ()
                                }
                                frame #1 {
                                n8016 = local read "Buffer-C2 Pumping\nResolution"() -> (w8433:T2)
                                n8017 = case shown="\"Standard Pumping\", Default" w8433 {
                                tunnel: [w8434 w8445] -> w8432
                                frame "Standard Pumping", Default {
                                n8018 = local read "Buffer-C2 Volume \nto be Pumped"() -> (w8437:dbl)
                                n8019 = local read "Volume of Syringe"() -> (w8440:dbl)
                                n8020 = local read "Initial Plunger Position"() -> (w8444:dbl)
                                n8021 = local read "Position\nNow"() -> (w8443:dbl)
                                n8022 = Subtract(x=w8444, y=w8443) -> (x-y=w8442:dbl)
                                n8023 = Absolute Value(x=w8442) -> (abs(x)=w8441:dbl)
                                n8024 = Multiply(x=w8441, y=w8440) -> (x*y=w8439:dbl)
                                n8025 = Divide(x=w8439, y=3000.0) -> (x/y=w8436:dbl)
                                n8026 = Subtract(x=w8436, y=w8437) -> (x-y=w8435:dbl)
                                n8027 = Absolute Value(x=w8435) -> (abs(x)=w8434:dbl)
                                }
                                frame "High Resolution Pumping" {
                                n8028 = local read "Buffer-C2 Volume \nto be Pumped"() -> (w8448:dbl)
                                n8029 = local read "Volume of Syringe"() -> (w8451:dbl)
                                n8030 = local read "Initial Plunger Position"() -> (w8455:dbl)
                                n8031 = local read "Position\nNow"() -> (w8454:dbl)
                                n8032 = Subtract(x=w8455, y=w8454) -> (x-y=w8453:dbl)
                                n8033 = Absolute Value(x=w8453) -> (abs(x)=w8452:dbl)
                                n8034 = Multiply(x=w8452, y=w8451) -> (x*y=w8450:dbl)
                                n8035 = Divide(x=w8450, y=24000.0) -> (x/y=w8447:dbl)
                                n8036 = Subtract(x=w8447, y=w8448) -> (x-y=w8446:dbl)
                                n8037 = Absolute Value(x=w8446) -> (abs(x)=w8445:dbl)
